vi "Do Insertion.vi"(6 "Last Insertion Time":timestamp, 8 "error in (no error)":errorcluster, 9 "View Name":string, 10 "VI Refnum":refnum<vi>, 11 "ProtectedSubpanel in":refnum<class "ProtectedSubpanel.lvclass">) -> (0 "error out":errorcluster, 3 "ProtectedSubpanel out":refnum<class "ProtectedSubpanel.lvclass">)   [LabVIEW 2015, in "ProtectedSubpanel.lvlib" / "ProtectedSubpanel.lvclass"]
uses:
  ProtectedSubpanel.lvclass
  ProtectedSubpanel.lvclass/ProtectedSubpanel.ctl
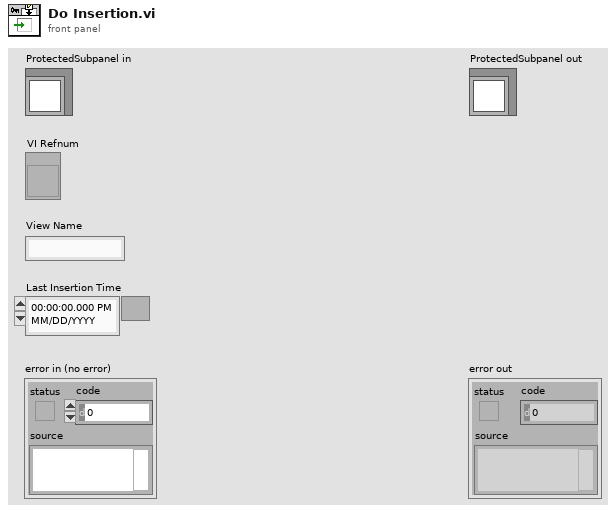
[diagram p1: front panel]
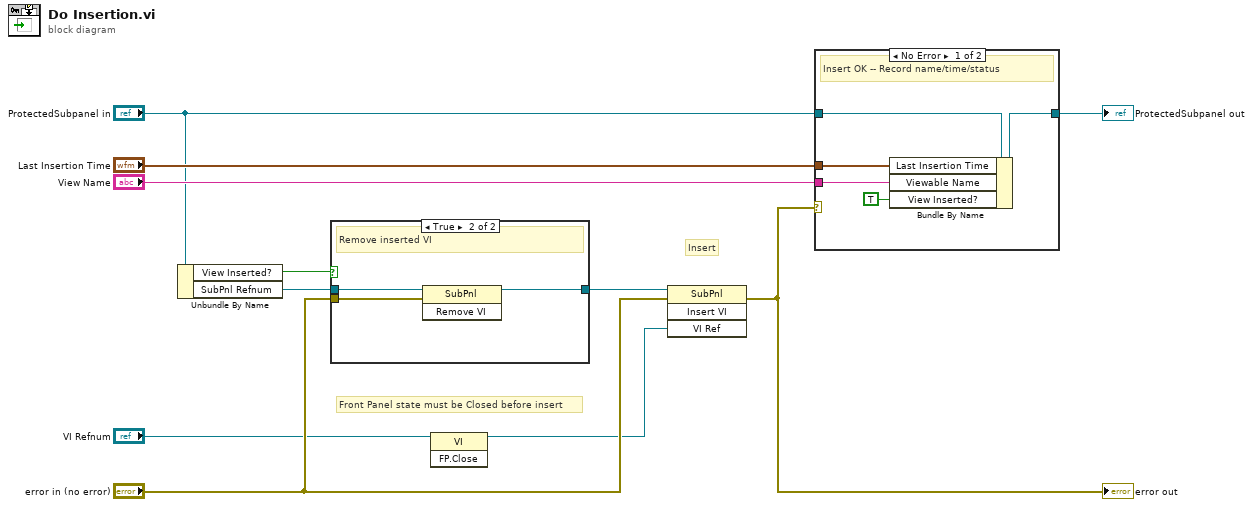
[diagram p0: block diagram]
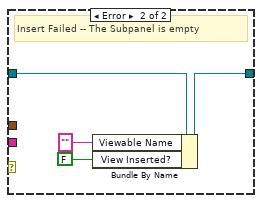
[diagram p2: hidden frame]
diagram:
  # "Front Panel state must be Closed before insert"
  # "Insert"
  n1 = Unbundle By Name("ProtectedSubpanel in") -> ("View Inserted?"=w10:bool, "SubPnl Refnum"=w11:refnum<vi>)
  n2 = case shown="True" w10 {
    tunnel: w11 -> [w12 w15]
    tunnel: "error in (no error)" -> [_ w14]
    tunnel: [w12 w13] -> w9
    frame False {
      # "Do nothing"
    }
    frame True {
      # "Remove inserted VI"
      n3 = invoke class="SubPnl" method="Remove VI"(reference=w15, error in=w14) -> (reference out=w13:refnum<vi>)  [unwired: 1 in, 2 out]
    }
  }
  n4 = invoke class="VI" method="FP.Close"(reference="VI Refnum") -> (reference out=w5:refnum<vi>)  [unwired: 2 in, 2 out]
  n5 = invoke class="SubPnl" method="Insert VI"(reference=w9, error in="error in (no error)", "VI Ref"=w5) -> (error out=w3:errorcluster)  [unwired: 1 in, 3 out]
  "error out" <- w3
  n6 = case shown="No Error" w3 {
    tunnel: [w20 w23] -> w8
    tunnel: "Last Insertion Time" -> [w19 _]
    tunnel: "ProtectedSubpanel in" -> [w18 w24]
    tunnel: "View Name" -> [w17 _]
    frame No Error {
      # "Insert OK -- Record name/time/status"
      n7 = Bundle By Name(cluster=w18, "Last Insertion Time"=w19, "Viewable Name"=w17, "View Inserted?"=TRUE) -> (w20:refnum<class "ProtectedSubpanel.lvclass">)
    }
    frame Error {
      # "Insert Failed -- The Subpanel is empty"
      n8 = Bundle By Name(cluster=w24, "Viewable Name"="" ("Inserted View Name"), "View Inserted?"=FALSE) -> (w23:refnum<class "ProtectedSubpanel.lvclass">)
    }
  }
  "ProtectedSubpanel out" <- w8
